vi "CheckDataCalculationValid.vi"(8 "Working Current":T2, 10 "Percent FLA Value":dbl, 11 "Channel Name":string) -> (1 "Motor State":T1, 2 ">min working current":bool, 3 "< max working current":bool)   [LabVIEW 2016, in "McsaAnalysisFunctions.lvlib"]
uses:
  <vilib>/addons/InsightCM/Utilities/Analysis/MCSA/McsaAnalysisFunctions.lvlib
  <vilib>/addons/InsightCM/Utilities/Analysis/MCSA/controls/WorkingCurrent.ctl
  <vilib>/addons/InsightCM/Utilities/Analysis/MCSA/controls/MotorState.ctl
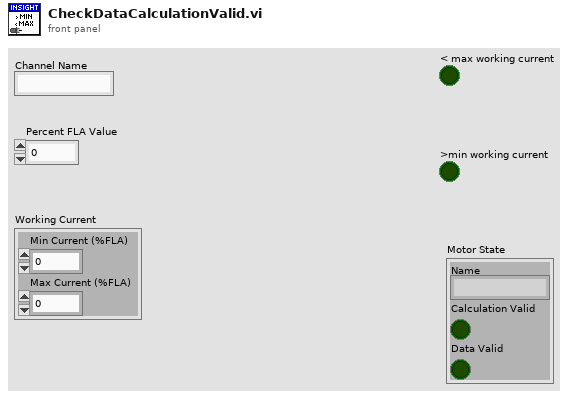
[diagram p1: front panel]
types:
  T1 = typedef "McsaAnalysisFunctions.lvlib/MotorState.ctl" = cluster{"Name":string, "Calculation Valid":bool, "Data Valid":bool}
  T2 = typedef "McsaAnalysisFunctions.lvlib/WorkingCurrent.ctl" = cluster{"Min Current (%FLA)":dbl, "Max Current (%FLA)":dbl}
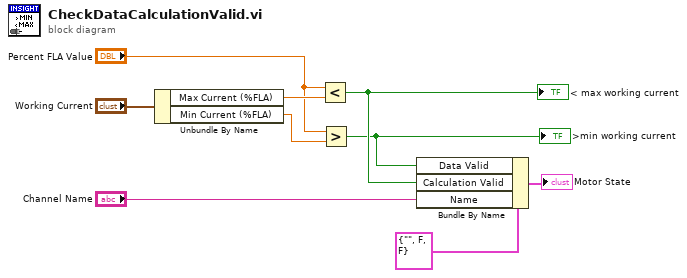
[diagram p0: block diagram]
diagram:
  n1 = Unbundle By Name("Working Current") -> ("Max Current (%FLA)"=w5:dbl, "Min Current (%FLA)"=w4:dbl)
  n2 = Less?(x="Percent FLA Value", y=w5) -> (x < y?=w2:bool)
  "< max working current" <- w2
  n3 = Greater?(x="Percent FLA Value", y=w4) -> (0:w1:bool)
  ">min working current" <- w1
  n4 = Bundle By Name(cluster=T1 {"Name"="", "Calculation Valid"=FALSE, "Data Valid"=FALSE} ("MCSA FFT"), "Data Valid"=w1, "Calculation Valid"=w2, "Name"="Channel Name") -> (→"Motor State":T1)
